vi "KB- Save Total Pass NG Number.vi"(10 "ParamSet":string[](array[string]), 11 "名称或相对路径":string="UserDefine.ini") -> ()   [LabVIEW 2015]
uses:
  Global System.vi
  <vilib>/Utility/config.llb/NI_LVConfig.lvlib
panel:
  in  "error in (no error)":errorcluster caption="错误输入（无错误）"
  out "error out":errorcluster caption="错误输出"
  out "添加的路径":path
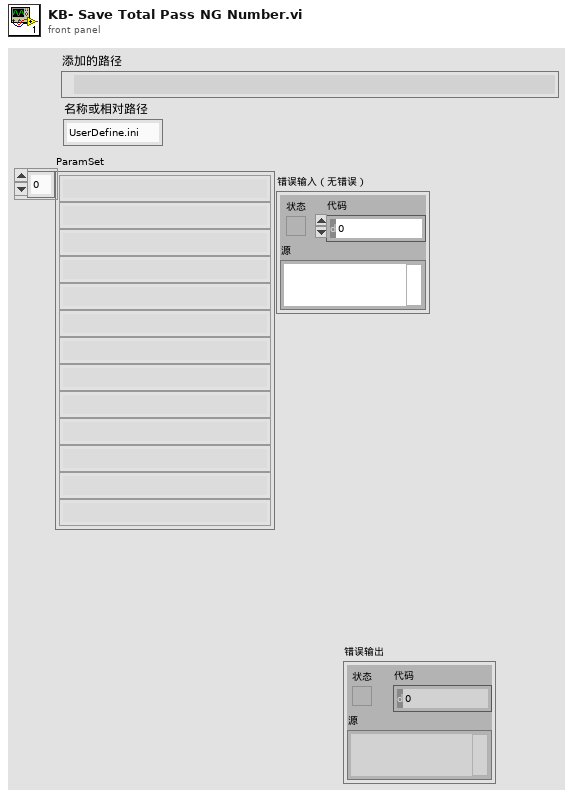
[diagram p1: front panel]
types:
  T1 = typedef "NI_LVConfig.lvlib/Config Data RefNum.ctl" = refnum<k1>
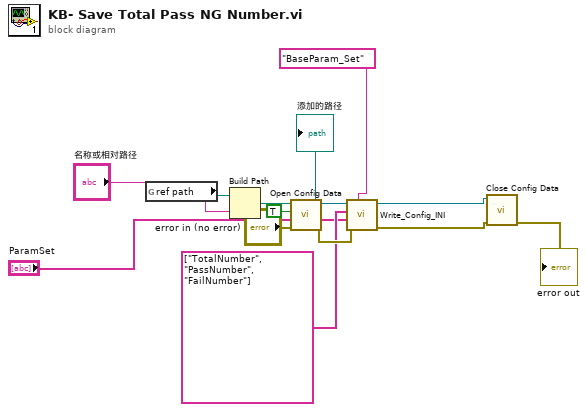
[diagram p0: block diagram]
diagram:
  n1 = global read "Global System.vi" "ref path"() -> (w7:path)
  n2 = Build Path(base path=w7, name or relative path="名称或相对路径") -> (appended path=w10:path)
  "添加的路径" <- w10
  n3 = call <vilib>:"Open Config Data.vi"("error in (no error)"="error in (no error)", "create file if necessary (T)"=TRUE, "configuration file path"=w10) -> ("error out"=w12:errorcluster, "refnum"=w11:T1)  [unwired: 6 in, 1 out]
  n4 = call "Write_Config_INI.vi"("section"="BaseParam_Set", "error in (no error)"=w12, "Inputs"="ParamSet", "Keys"=string[] ["TotalNumber", "PassNumber", "FailNumber"], "refnum"=w11) -> ("error out"=w3:errorcluster, "refnum 2"=w4:T1)  [unwired: 5 in]
  n5 = call <vilib>:"Close Config Data.vi"("error in (no error)"=w3, "refnum"=w4) -> ("error out"=→"error out":errorcluster)  [unwired: 8 in, 1 out]
